vi "set entype settings.vi"(8 "error in (no error)":errorcluster, 10 "entype_settings":cluster{"EngineType":u32, "DriverType":u32}, 11 "id":i32) -> (0 "error out":errorcluster, 3 "function return":i32)   [LabVIEW 2012, in "libximc.lvlib"]
doc: "result_t XIMC_API set_entype_settings (device_t id, const entype_settings_t* entype_settings);"
uses:
  libximc.lvlib
  libximc.dll
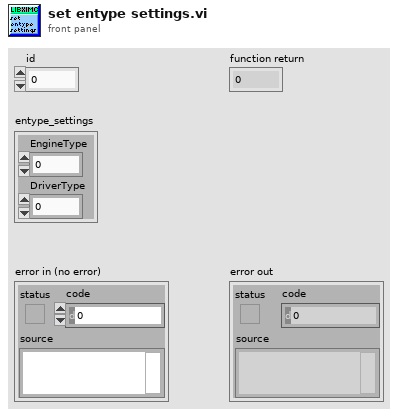
[diagram p1: front panel]
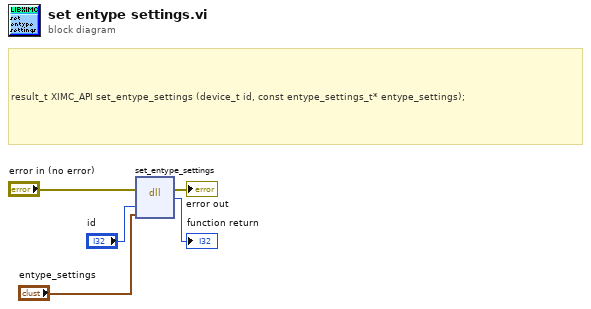
[diagram p0: block diagram]
diagram:
  # "result_t XIMC_API set_entype_settings (device_t id, const entype_settings_t* entype_settings);"
  n1 = dll-call lib="C:/Users/Vasily/Att_examples/LabVIEW_example/libximc.*" fn="set_entype_settings"(error in="error in (no error)", "id"="id", "entype_settings"="entype_settings") -> (error out=→"error out":errorcluster, →"function return":i32)  [unwired: 4 in, 1 out]
